vi "SDCP - Standard Message Frames Editor - Generate Parameter File.vi"(2 "error in (no error)":errorcluster, 3 "Frame details":T2(array[cluster])) -> (0 "error out":errorcluster, 1 "Output":string)   [LabVIEW 2020]
uses:
  Typedefs/SDCP - Standard Message Frames Editor - Parameter cluster.ctl
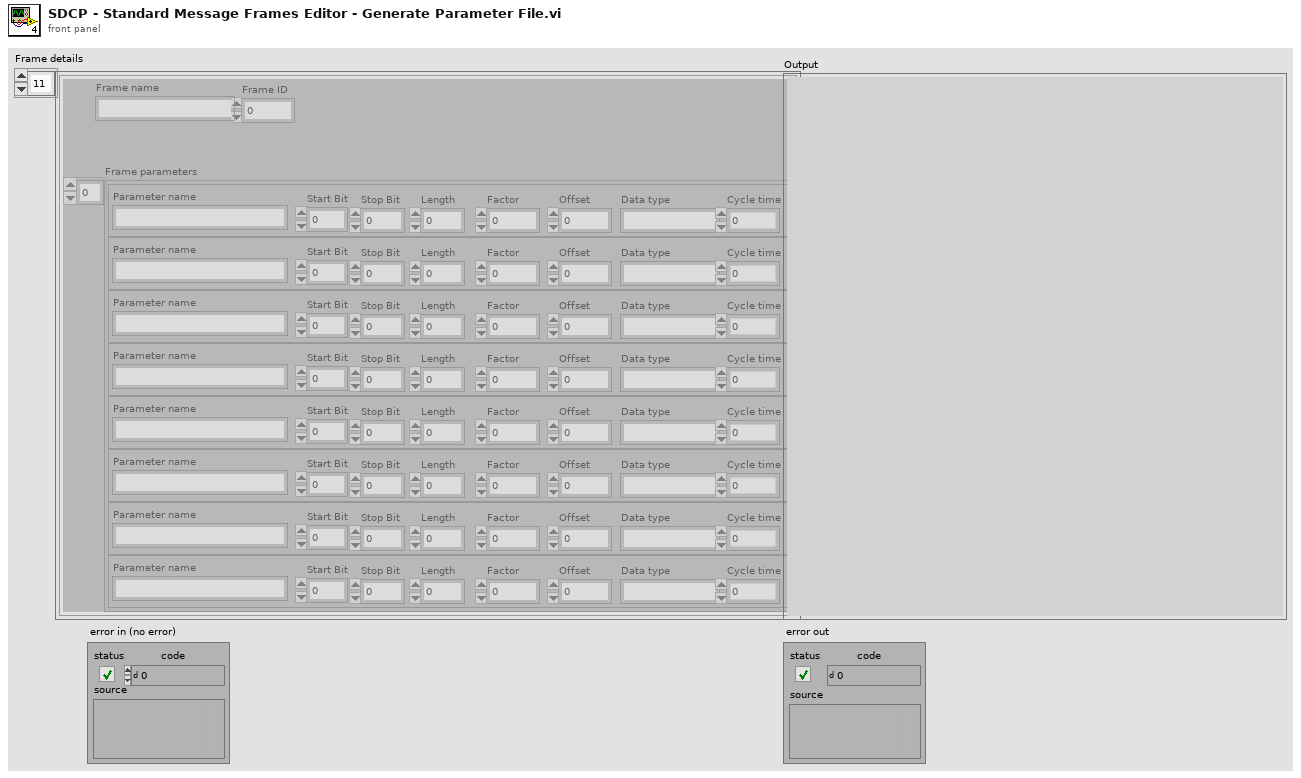
[diagram p1: front panel]
types:
  T1 = typedef "SDCP - Standard Message Frames Editor - Parameter cluster.ctl" = cluster{"Parameter name":string, "Start Bit":i32, "Stop Bit":i32, "Length":i32, "Factor":dbl, "Offset":dbl, "Data type":string, "Cycle time":dbl}
  T2 = cluster{"Frame name":string, "Frame ID":i32, "Frame parameters":T1[]}[]
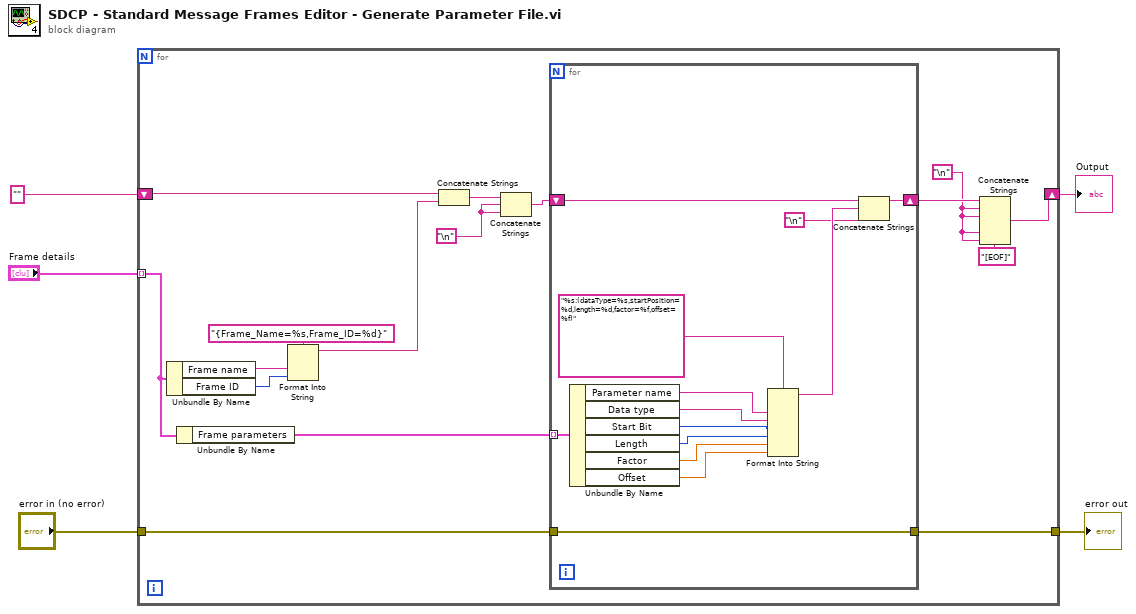
[diagram p0: block diagram]
diagram:
  n1 = for {
    tunnel: "Frame details" -> [w13] mode=indexing
    shift-right: [w8] -> w1
    shift-left: "" -> [w18]
    tunnel: "error in (no error)" -> [w15]
    tunnel: [w11] -> w2
    w6 = "\n"
    w10 = "\n"
    n2 = Unbundle By Name(w13) -> ("Frame name"=w20:string, "Frame ID"=w19:i32)
    n3 = Unbundle By Name(w13) -> ("Frame parameters"=w12:T1[])
    n4 = Format Into String(format string="{Frame_Name=%s,Frame_ID=%d}", w20, w19) -> (resulting string=w17:string)  [unwired: 2 in, 1 out]
    n5 = Concatenate Strings(w18, w17) -> (w16:string)
    n6 = Concatenate Strings(w16, w10, w10) -> (w14:string)
    n7 = for {
      tunnel: w15 -> [w26]
      shift-right: [w23] -> w9
      shift-left: w14 -> [w25]
      tunnel: w12 -> [w34] mode=indexing
      tunnel: [w26] -> w11
      n8 = Unbundle By Name(w34) -> ("Parameter name"=w32:string, "Data type"=w31:string, "Start Bit"=w30:i32, "Length"=w29:i32, "Factor"=w28:dbl, "Offset"=w27:dbl)
      n9 = Format Into String(format string="%s:(dataType=%s,startPosition=%d,length=%d,factor=%f,offset=%f)", w32, w31, w30, w29, w28, w27) -> (resulting string=w24:string)  [unwired: 2 in, 1 out]
      n10 = Concatenate Strings(w25, w24, "\n") -> (w23:string)
    }
    n11 = Concatenate Strings(w9, w6, w6, "[EOF]" ("string"), w6, w6) -> (w8:string)
  }
  "error out" <- w2
  "Output" <- w1
